vi "CheckAllowEdit.vi"(9 "点":T1, 10 "ref in":refnum<vi>) -> ()   [LabVIEW 2016]
uses:
  <vilib>/Utility/miscctls.llb/LVPositionTypeDef.ctl
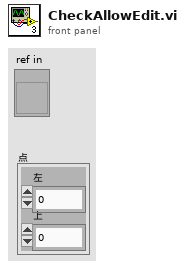
[diagram p1: front panel]
types:
  T1 = typedef "LVPositionTypeDef.ctl" = cluster{"Left":i32, "Top":i32}
  T2 = typedef "LVRowAndColumnTypeDef.ctl" = cluster{"Row":i32, "Column":i32}
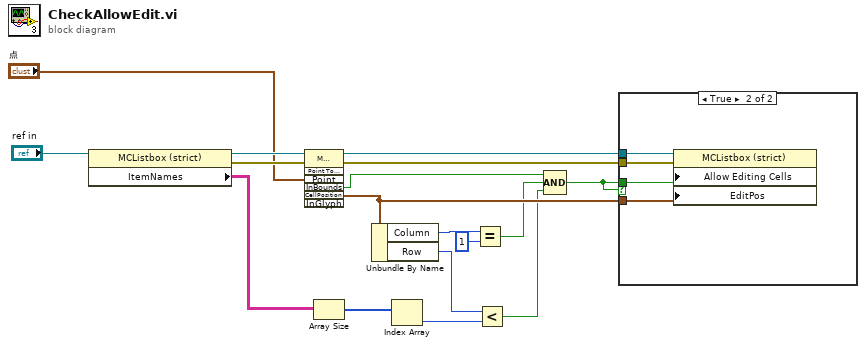
[diagram p0: block diagram]
diagram:
  n1 = property class="MCListbox (strict)"(reference="ref in") -> (reference out=w9:refnum<vi>, error out=w8:errorcluster, "ItemNames"=w7:string[][])  [unwired: 1 in]
  n2 = invoke class="MCListbox (严格)" method="Point To Row Column"(reference=w9, error in=w8, "Point"="点") -> (reference out=w15:refnum<vi>, error out=w11:errorcluster, "InBounds"=w13:bool, "CellPosition"=w14:T2)  [unwired: 4 in, 3 out]
  n3 = Array Size(array=w7) -> (size(s)=w6:i32[])
  n4 = Unbundle By Name(w14) -> ("Column"=w17:i32, "Row"=w5:i32)
  n5 = Index Array(array=w6) -> (element=w4:i32)  [unwired: 1 in]
  n6 = Equal?(x=w17, y=1) -> (x = y?=w12:bool)
  n7 = Less?(x=w5, y=w4) -> (x < y?=w3:bool)
  n8 = Compound Arithmetic op=AND(w13, w12, w3) -> (w2:bool)
  n9 = case shown="True" w2 {
    tunnel: w15 -> [_ w21]
    tunnel: w14 -> [_ w20]
    tunnel: w2 -> [_ w19]
    tunnel: w11 -> [_ w18]
    frame False {
    }
    frame True {
      n10 = property on="属性节点" class="MCListbox (strict)"(reference=w21, error in=w18, "Allow Editing Cells"=w19, "EditPos"=w20) -> ()  [unwired: 2 out]
    }
  }
